vi "Amplitude.vi"(7 "LabVIEW Web Service Request":refnum<class "Web Request.lvclass">) -> ()   [LabVIEW 2023]
uses:
  <vilib>/wsapi/Web Request.lvclass
panel:
  # "Use the Web Service Request input terminal to call the VIs on the Web Services palette. Do not remove it from the connector pane unless you don't need access to the palette."
  # "Each additional control wired to the connector pane will be available as an input in the URL. To include an indicator in terminal-mode output (the default setting), it must also be wired to the connector pane."
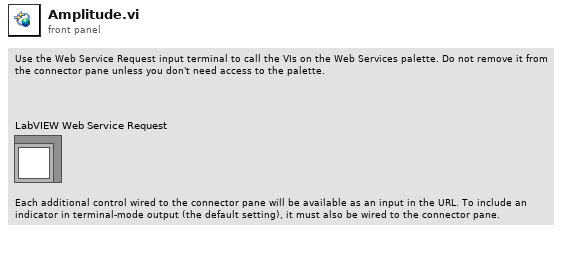
[diagram p1: front panel]
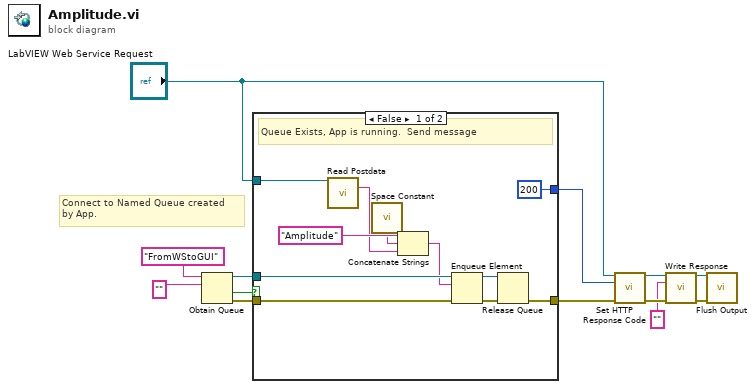
[diagram p0: block diagram]
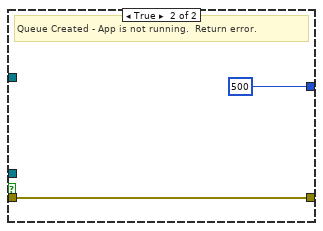
[diagram p2: hidden frame]
diagram:
  # "Connect to Named Queue created\nby App."
  n1 = Obtain Queue(name (unnamed)="FromWStoGUI", element data type="") -> (queue out=w10:refnum<queue>, created new?=w11:bool, error out=w9:errorcluster)  [unwired: 3 in]
  n2 = case shown="False" w11 {
    tunnel: w10 -> [w24 _]
    tunnel: w9 -> [w23 w26]
    tunnel: [w20 w26] -> w8
    tunnel: [200 500] -> w7
    tunnel: "LabVIEW Web Service Request" -> [w18 _]
    frame False {
      # "Queue Exists, App is running.  Send message"
      n3 = call <vilib>:"Read Postdata.vi"("LabVIEW Web Service Request"=w18) -> ("postdata"=w16:string)  [unwired: 12 in, 2 out]
      n4 = call <vilib>:"Space Constant.vi"() -> ("String"=w15:string)
      n5 = Concatenate Strings("Amplitude", w15, w16) -> (w14:string)
      n6 = Enqueue Element(queue=w24, element=w14, error in (no error)=w23) -> (queue out=w22:refnum<queue>, error out=w21:errorcluster)  [unwired: 1 in, 1 out]
      n7 = Release Queue(queue=w22, error in (no error)=w21) -> (error out=w20:errorcluster)  [unwired: 1 in, 2 out]
    }
    frame True {
      # "Queue Created - App is not running.  Return error."
    }
  }
  n8 = call <vilib>:"Set HTTP Response Code.vi"("LabVIEW Web Service Request"="LabVIEW Web Service Request", "response code (200)"=w7, "error in (no error)"=w8) -> ("LabVIEW Web Service Request out"=w6:refnum<class "Web Request.lvclass">, "error out"=w5:errorcluster)  [unwired: 11 in]
  n9 = call <vilib>:"Write Response.vi"("LabVIEW Web Service Request"=w6, "response string"="", "error in (no error)"=w5) -> ("LabVIEW Web Service Request out"=w3:refnum<class "Web Request.lvclass">, "error out"=w2:errorcluster)  [unwired: 11 in]
  n10 = call <vilib>:"Flush Output.vi"("LabVIEW Web Service Request"=w3, "error in (no error)"=w2) -> ()  [unwired: 12 in, 2 out]
